vi "BC RT Main.vi"() -> ()   [LabVIEW 2020]
panel:
  out "Timeout Length":i32
  out "AO Error":errorcluster
  out "Status?":string
  out "Diagnostics":string
  out "Keg Level":u8(slide) scale=0.0..100.0
  out "Pouring...":u8(slide) scale=0.0..100.0
  in  "24 Oz":bool
  in  "16 Oz":bool
  in  "12 Oz":bool
  in  "Cancel Pour":bool
  in  "Stop":bool
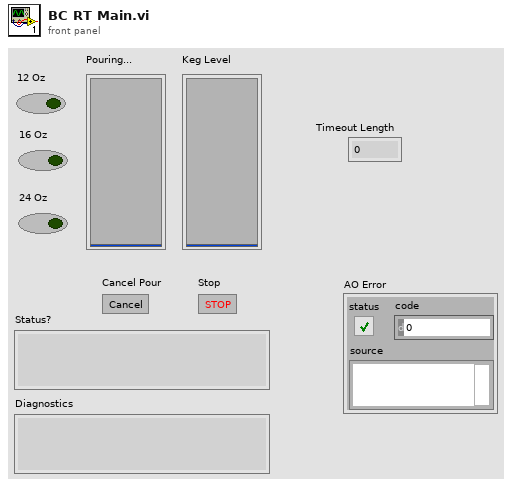
[diagram p1: front panel]
types:
  T1 = cluster{"Stop":refnum<user-event>, "Cancel":refnum<user-event>, "Pour":refnum<user-event>}
  T2 = cluster{"Status?":refnum<vi>, "Stop":refnum<vi>, "Diagnostics":refnum<vi>, "Keg Level":refnum<vi>, "Pouring...":refnum<vi>, "24 Oz":refnum<vi>, "16 Oz":refnum<vi>, "12 Oz":refnum<vi>, "Cancel Pour":refnum<vi>}
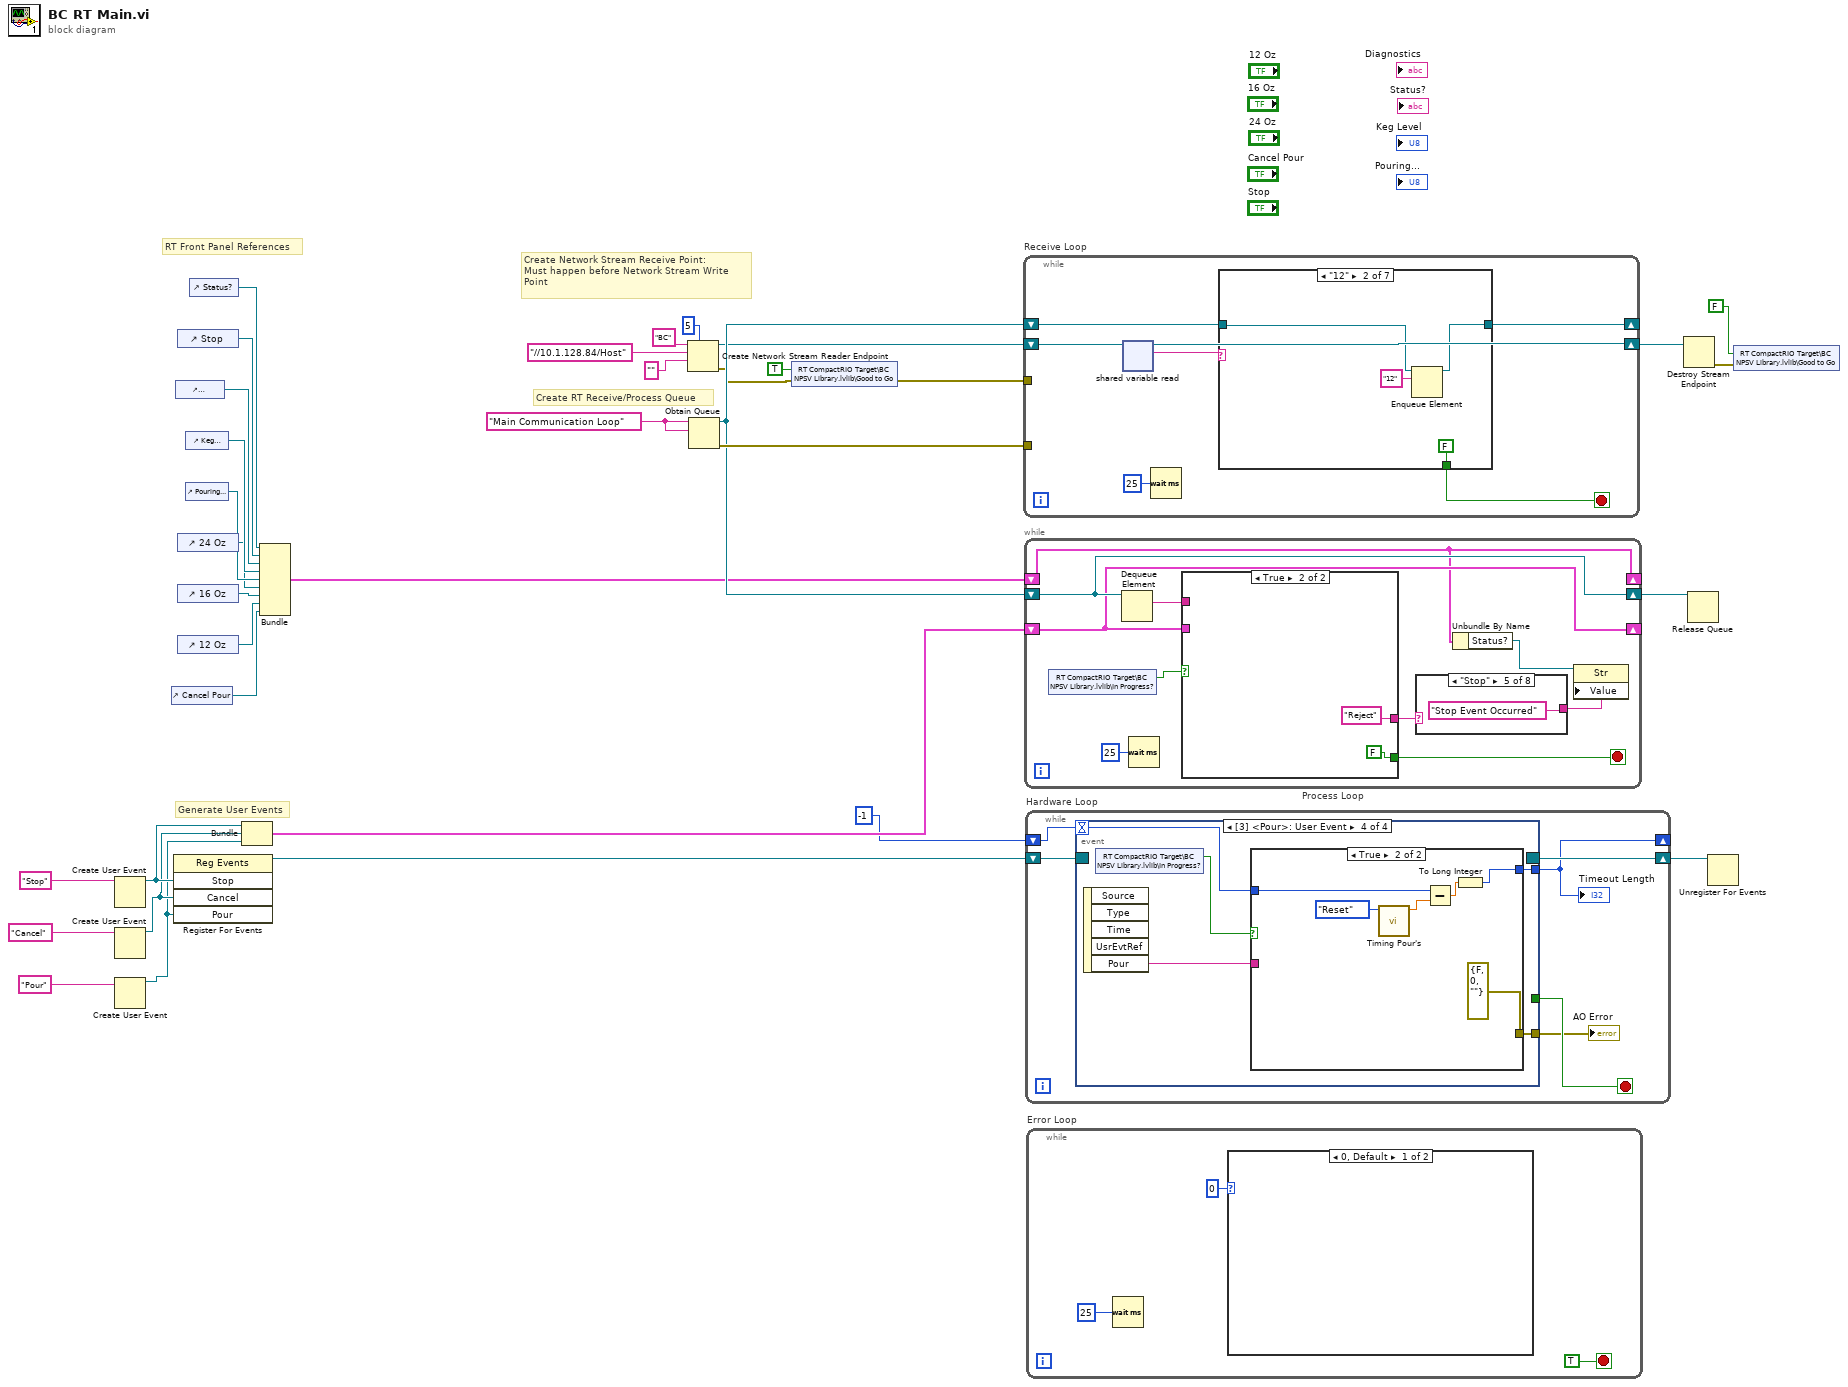
[diagram p0: block diagram]
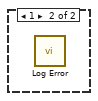
[diagram p2: hidden frame]
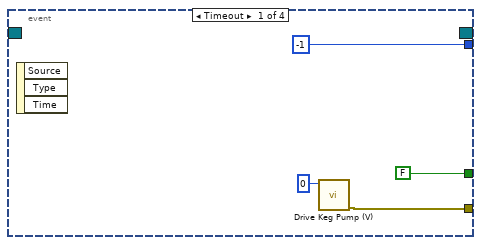
[diagram p3: hidden frame]
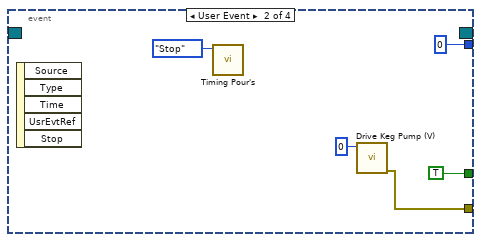
[diagram p4: hidden frame]
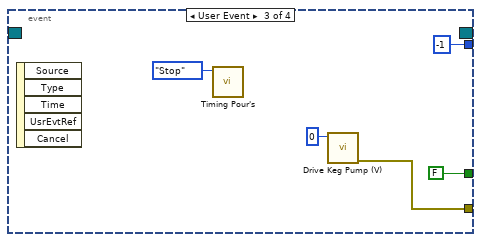
[diagram p5: hidden frame]
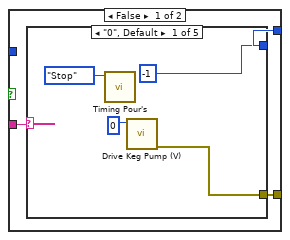
[diagram p6: hidden frame]
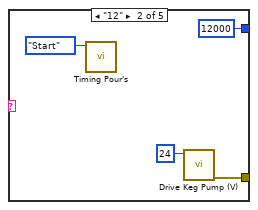
[diagram p7: hidden frame]
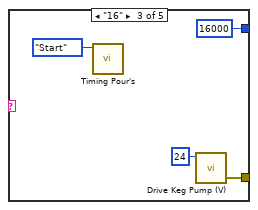
[diagram p8: hidden frame]
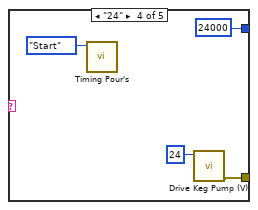
[diagram p9: hidden frame]
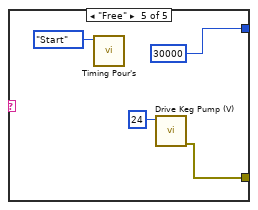
[diagram p10: hidden frame]
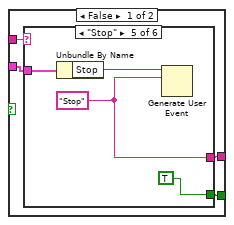
[diagram p11: hidden frame]
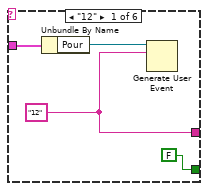
[diagram p12: hidden frame]
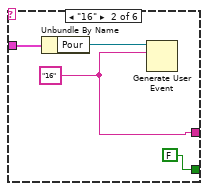
[diagram p13: hidden frame]
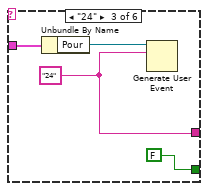
[diagram p14: hidden frame]
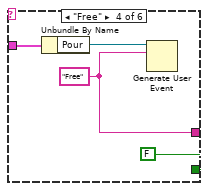
[diagram p15: hidden frame]
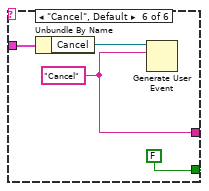
[diagram p16: hidden frame]
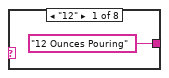
[diagram p17: hidden frame]
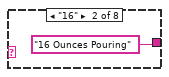
[diagram p18: hidden frame]
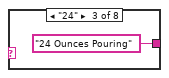
[diagram p19: hidden frame]
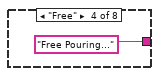
[diagram p20: hidden frame]
diagram:
  w7 = "Main Communication Loop" ("name (unnamed)")
  # "Create RT Receive/Process Queue"
  # "Create Network Stream Receive Point:\nMust happen before Network Stream Write\nPoint"
  # "RT Front Panel References"
  # "Generate User Events"
  n1 = Create User Event(user event datatype="Stop" ("Stop")) -> (user event=w13:refnum<user-event>)  [unwired: 1 in, 1 out]
  n2 = Create User Event(user event datatype="Cancel" ("Cancel")) -> (user event=w12:refnum<user-event>)  [unwired: 1 in, 1 out]
  n3 = Create User Event(user event datatype="Pour" ("Pour")) -> (user event=w11:refnum<user-event>)  [unwired: 1 in, 1 out]
  n4 = control-ref of="Cancel Pour"() -> (w26:refnum<vi>)
  n5 = register-events(w13, w12, w11) -> (reference out=w14:refnum<event-registration>)  [unwired: 2 in, 1 out]
  n6 = control-ref of="Diagnostics"() -> (w32:refnum<vi>)
  n7 = control-ref of="Stop"() -> (w33:refnum<vi>)
  n8 = control-ref of="24 Oz"() -> (w29:refnum<vi>)
  n9 = control-ref of="16 Oz"() -> (w28:refnum<vi>)
  n10 = control-ref of="12 Oz"() -> (w27:refnum<vi>)
  n11 = control-ref of="Keg Level"() -> (w31:refnum<vi>)
  n12 = control-ref of="Pouring..."() -> (w30:refnum<vi>)
  n13 = control-ref of="Status?"() -> (w34:refnum<vi>)
  n14 = Bundle("Stop"=w13, "Cancel"=w12, "Pour"=w11) -> (w10:T1)  [unwired: 1 in]
  n15 = Bundle("Status?"=w34, "Stop"=w33, "Diagnostics"=w32, "Keg Level"=w31, "Pouring..."=w30, "24 Oz"=w29, "16 Oz"=w28, "12 Oz"=w27, "Cancel Pour"=w26) -> (w24:T2)  [unwired: 1 in]
  n16 = Create Network Stream Reader Endpoint(7:5 ("reader buffer size"), 9:"" ("writer url"), 10:"//10.1.128.84/Host" ("writer url"), 11:"BC" ("reader name")) -> (0:w4:errorcluster, 3:w23:refnum<k21>)  [unwired: 3 in]
  n17 = Obtain Queue(name (unnamed)=w7, element data type=w7) -> (queue out=w25:refnum<queue>, error out=w35:errorcluster)  [unwired: 3 in, 1 out]
  n18 = shared-variable "RT CompactRIO Target\\BC NPSV Library.lvlib\\Good to Go"(TRUE ("Good to Go"), error in=w4) -> (error out=w1:errorcluster)
  n19 = while "Receive Loop" {
    tunnel: w35 -> [_]
    shift-right: [w41] -> _
    shift-left: w25 -> [w42]
    shift-right: [w39] -> w22
    shift-left: w23 -> [w40]
    tunnel: w1 -> [_]
    stop <- w37 stop-if-true
    n20 = shared-variable-read(w40) -> (w39:refnum<k21>, w38:string)  [unwired: 2 in, 2 out]
    n21 = Wait (ms)(milliseconds to wait=u32 25) -> ()  [unwired: 1 out]
    n22 = case shown="\"12\"" w38 {
      tunnel: w42 -> [w46 w50 w54 w58 w62 w64 w69]
      tunnel: [w45 w49 w53 w57 w61 w67 w72] -> w41
      tunnel: [FALSE FALSE FALSE FALSE FALSE FALSE TRUE] -> w37
      frame "0", Default {
        n23 = Enqueue Element(queue=w46, element="0") -> (queue out=w45:refnum<queue>)  [unwired: 2 in, 2 out]
      }
      frame "12" {
        n24 = Enqueue Element(queue=w50, element="12") -> (queue out=w49:refnum<queue>)  [unwired: 2 in, 2 out]
      }
      frame "16" {
        n25 = Enqueue Element(queue=w54, element="16") -> (queue out=w53:refnum<queue>)  [unwired: 2 in, 2 out]
      }
      frame "24" {
        n26 = Enqueue Element(queue=w58, element="24") -> (queue out=w57:refnum<queue>)  [unwired: 2 in, 2 out]
      }
      frame "Free" {
        n27 = Enqueue Element(queue=w62, element="Free") -> (queue out=w61:refnum<queue>)  [unwired: 2 in, 2 out]
      }
      frame "Cancel" {
        n28 = Flush Queue(queue=w64) -> (queue out=w63:refnum<queue>)  [unwired: 1 in, 2 out]
        n29 = Enqueue Element(queue=w63, element="Cancel") -> (queue out=w67:refnum<queue>)  [unwired: 2 in, 2 out]
      }
      frame "Stop" {
        n30 = Flush Queue(queue=w69) -> (queue out=w68:refnum<queue>)  [unwired: 1 in, 2 out]
        n31 = Enqueue Element(queue=w68, element="Stop") -> (queue out=w72:refnum<queue>)  [unwired: 2 in, 2 out]
      }
    }
  }
  n32 = while "Process Loop" {
    shift-right: [w78] -> _
    shift-left: w10 -> [w78]
    shift-right: [w79] -> w8
    shift-left: w25 -> [w79]
    shift-right: [w74] -> _
    shift-left: w24 -> [w74]
    stop <- w81 stop-if-true
    n33 = shared-variable "RT CompactRIO Target\\BC NPSV Library.lvlib\\In Progress?"() -> (w75:bool)  [unwired: 1 in, 1 out]
    n34 = Dequeue Element(queue=w79) -> (element=w82:string)  [unwired: 2 in, 3 out]
    n35 = Wait (ms)(milliseconds to wait=u32 25) -> ()  [unwired: 1 out]
    n36 = case shown="True" w75 {
      tunnel: w82 -> [w86 _]
      tunnel: [w85 FALSE] -> w81
      tunnel: w78 -> [w84 _]
      tunnel: [w83 "Reject" ("Stop")] -> w76
      frame False {
        n37 = case shown="\"Stop\"" w86 {
          tunnel: [FALSE FALSE FALSE FALSE TRUE FALSE] -> w85
          tunnel: w84 -> [w89 w93 w97 w101 w105 w108]
          tunnel: [w87 w91 w95 w99 w104 w107] -> w83
          frame "12" {
            w87 = "12" ("Stop")
            n38 = Unbundle By Name(w89) -> ("Pour"=w90:refnum<user-event>)
            n39 = Generate User Event(user event=w90, event data cluster=w87) -> ()  [unwired: 2 in, 2 out]
          }
          frame "16" {
            w91 = "16" ("Stop")
            n40 = Unbundle By Name(w93) -> ("Pour"=w94:refnum<user-event>)
            n41 = Generate User Event(user event=w94, event data cluster=w91) -> ()  [unwired: 2 in, 2 out]
          }
          frame "24" {
            w95 = "24" ("Stop")
            n42 = Unbundle By Name(w97) -> ("Pour"=w98:refnum<user-event>)
            n43 = Generate User Event(user event=w98, event data cluster=w95) -> ()  [unwired: 2 in, 2 out]
          }
          frame "Free" {
            w99 = "Free" ("Stop")
            n44 = Unbundle By Name(w101) -> ("Pour"=w102:refnum<user-event>)
            n45 = Generate User Event(user event=w102, event data cluster=w99) -> ()  [unwired: 2 in, 2 out]
          }
          frame "Stop" {
            w104 = "Stop" ("Stop")
            n46 = Unbundle By Name(w105) -> ("Stop"=w106:refnum<user-event>)
            n47 = Generate User Event(user event=w106, event data cluster=w104) -> ()  [unwired: 2 in, 2 out]
          }
          frame "Cancel", Default {
            w107 = "Cancel" ("Stop")
            n48 = Unbundle By Name(w108) -> ("Cancel"=w110:refnum<user-event>)
            n49 = Generate User Event(user event=w110, event data cluster=w107) -> ()  [unwired: 2 in, 2 out]
          }
        }
      }
      frame True {
      }
    }
    n50 = case shown="\"Stop\"" w76 {
      tunnel: ["12 Ounces Pouring" "16 Ounces Pouring" "24 Ounces Pouring" "Free Pouring..." "Stop Event Occurred" ("Cancel") "Pour Canceled" ("Cancel") "Pour Canceled" ("Cancel") "Pour Request Rejected..."] -> w77
      frame "12" {
      }
      frame "16" {
      }
      frame "24" {
      }
      frame "Free" {
      }
      frame "Stop" {
      }
      frame "Cancel", Default {
      }
      frame "Reject " {
      }
      frame "Reject" {
      }
    }
    n51 = Unbundle By Name(w74) -> ("Status?"=w73:refnum<vi>)
    n52 = property class="Str"(reference=w73, "Value"=w77) -> ()  [unwired: 1 in, 2 out]
  }
  n53 = while "Hardware Loop" {
    shift-right: [w125] -> w18
    shift-left: w14 -> [w124]
    shift-right: [w123] -> _
    shift-left: -1 -> [w121]
    stop <- w126 stop-if-true
    n54 = event shown="[3] <Pour>: User Event" {
      selector: w124 -> [_ _ _ _]
      dyn-events: [_ _ _ _] -> w125
      timeout: w121 -> [_ _ _ w142]
      tunnel: [FALSE TRUE FALSE _] -> w126
      tunnel: [-1 0 -1 w144] -> w123
      tunnel: [w127 w133 w137 w143] -> w122
      event Timeout {
        n55 = event-data() -> ()  [unwired: 1 in, 3 out]
        n56 = call "Drive Keg Pump (V).vi"("Voltage Select"=0) -> ("AO Error Out"=w127:errorcluster)  [unwired: 10 in]
      }
      event User Event {
        n57 = event-data() -> ()  [unwired: 1 in, 5 out]
        n58 = call "Timing Pour's.vi"("Timing Command"=enum16{"Reset", "Stop", "Start"}."Stop") -> ()  [unwired: 8 in, 3 out]
        n59 = call "Drive Keg Pump (V).vi"("Voltage Select"=0) -> ("AO Error Out"=w133:errorcluster)  [unwired: 10 in]
      }
      event User Event {
        n60 = event-data() -> ()  [unwired: 1 in, 5 out]
        n61 = call "Timing Pour's.vi"("Timing Command"=enum16{"Reset", "Stop", "Start"}."Stop") -> ()  [unwired: 8 in, 3 out]
        n62 = call "Drive Keg Pump (V).vi"("Voltage Select"=0) -> ("AO Error Out"=w137:errorcluster)  [unwired: 10 in]
      }
      event User Event {
        n63 = event-data() -> ("Pour"=w145:string)  [unwired: 1 in, 4 out]
        n64 = shared-variable "RT CompactRIO Target\\BC NPSV Library.lvlib\\In Progress?"() -> (w141:bool)  [unwired: 1 in, 1 out]
        n65 = case shown="True" w141 {
          tunnel: w145 -> [w148 _]
          tunnel: [w147 w170] -> w144
          tunnel: [w146 errorcluster {"status"=FALSE, "code"=0, "source"=""} ("AO Error Out")] -> w143
          tunnel: w142 -> [_ w171]
          frame False {
            n66 = case shown="\"0\", Default" w148 {
              tunnel: [-1 12000 16000 24000 30000] -> w147
              tunnel: [w150 w154 w159 w163 w166] -> w146
              frame "0", Default {
                n67 = call "Timing Pour's.vi"("Timing Command"=enum16{"Reset", "Stop", "Start"}."Stop") -> ()  [unwired: 8 in, 3 out]
                n68 = call "Drive Keg Pump (V).vi"("Voltage Select"=0) -> ("AO Error Out"=w150:errorcluster)  [unwired: 10 in]
              }
              frame "12" {
                n69 = call "Timing Pour's.vi"("Timing Command"=enum16{"Reset", "Stop", "Start"}."Start") -> ()  [unwired: 8 in, 3 out]
                n70 = call "Drive Keg Pump (V).vi"("Voltage Select"=24) -> ("AO Error Out"=w154:errorcluster)  [unwired: 10 in]
              }
              frame "16" {
                n71 = call "Timing Pour's.vi"("Timing Command"=enum16{"Reset", "Stop", "Start"}."Start") -> ()  [unwired: 8 in, 3 out]
                n72 = call "Drive Keg Pump (V).vi"("Voltage Select"=24) -> ("AO Error Out"=w159:errorcluster)  [unwired: 10 in]
              }
              frame "24" {
                n73 = call "Timing Pour's.vi"("Timing Command"=enum16{"Reset", "Stop", "Start"}."Start") -> ()  [unwired: 8 in, 3 out]
                n74 = call "Drive Keg Pump (V).vi"("Voltage Select"=24) -> ("AO Error Out"=w163:errorcluster)  [unwired: 10 in]
              }
              frame "Free" {
                n75 = call "Timing Pour's.vi"("Timing Command"=enum16{"Reset", "Stop", "Start"}."Start") -> ()  [unwired: 8 in, 3 out]
                n76 = call "Drive Keg Pump (V).vi"("Voltage Select"=24) -> ("AO Error Out"=w166:errorcluster)  [unwired: 10 in]
              }
            }
          }
          frame True {
            n77 = call "Timing Pour's.vi"("Timing Command"=enum16{"Reset", "Stop", "Start"}."Reset") -> ("Seconds Passed"=w172:dbl)  [unwired: 8 in, 2 out]
            n78 = Subtract(x=w171, y=w172) -> (x-y=w169:dbl)
            n79 = To Long Integer(number=w169) -> (32bit integer=w170:i32)
          }
        }
      }
    }
    "AO Error" <- w122
    "Timeout Length" <- w123
  }
  n80 = while "Error Loop" {
    stop <- TRUE stop-if-true
    n81 = Wait (ms)(milliseconds to wait=u32 25) -> ()  [unwired: 1 out]
    n82 = case shown="0, Default" 0 ("Int32") {
      frame 0, Default {
      }
      frame 1 {
        n83 = call "Log Error.vi"() -> ()  [unwired: 12 in]
      }
    }
  }
  n84 = Destroy Stream Endpoint(11:w22) -> (0:w2:errorcluster)  [unwired: 1 in]
  n85 = Release Queue(queue=w8) -> ()  [unwired: 2 in, 3 out]
  n86 = Unregister For Events(event registration refnum=w18) -> ()  [unwired: 1 in, 1 out]
  n87 = shared-variable "RT CompactRIO Target\\BC NPSV Library.lvlib\\Good to Go"(FALSE ("Good to Go"), error in=w2) -> ()  [unwired: 1 out]
